vi "Init MemberTable.vi"(8 "error in (no error)":errorcluster, 9 "SheetName(\"\")":string, 10 "Path":path, 11 "TimeTable in":refnum<class "TimeTable.lvclass">) -> (0 "error out":errorcluster, 3 "TimeTable out":refnum<class "TimeTable.lvclass">)   [LabVIEW 2015, in "Member_Actor.lvlib" / "TimeTable.lvclass"]
uses:
  TimeTable.lvclass
  TimeTable.lvclass/TimeTable.ctl
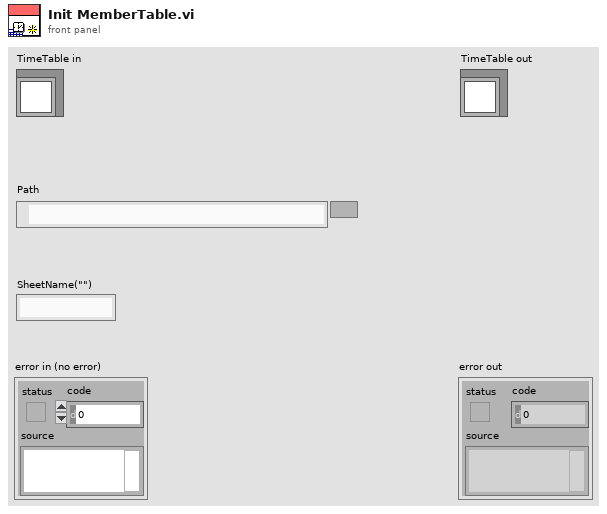
[diagram p1: front panel]
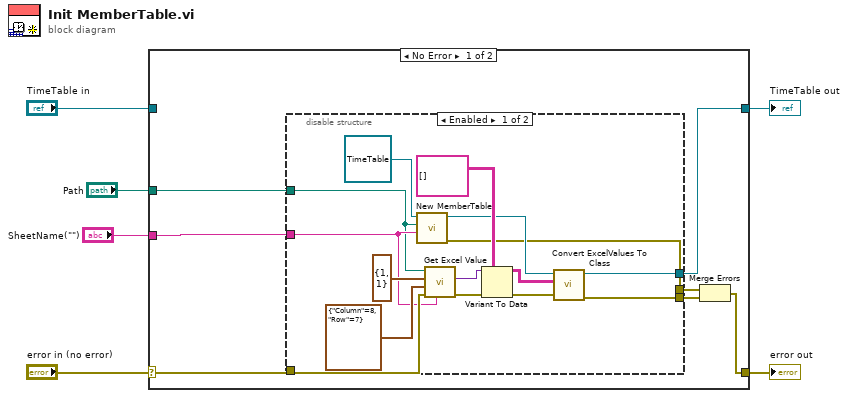
[diagram p0: block diagram]
diagram:
  n1 = case shown="No Error" "error in (no error)" {
    selector: "error in (no error)" -> [w10 w30]
    tunnel: [w12 w30] -> w5
    tunnel: [w11 w29] -> w3
    tunnel: "TimeTable in" -> [_ w29]
    tunnel: "Path" -> [w8 _]
    tunnel: "SheetName(\"\")" -> [w9 _]
    frame No Error {
      n2 = disable-structure shown="Enabled" {
        disable-tunnel: [w28 _] -> w13
        disable-tunnel: [w27 _] -> w11
        disable-tunnel: w10 -> [w20 _]
        disable-tunnel: w9 -> [w16 _]
        disable-tunnel: w8 -> [w15 _]
        disable-tunnel: [w14 _] -> w7
        frame Enabled {
          n3 = call "New MemberTable.vi"("SheetName(\"\")"=w16, "Path"=w15, "MemberTable in"=refnum<class "TimeTable.lvclass"> refnum) -> ("error out"=w14:errorcluster, "MemberTable out"=w17:refnum<class "TimeTable.lvclass">)  [unwired: 7 in]
          n4 = call "Get Excel Value.vi"("SheetName(\"\")"=w16, "error in (no error)"=w20, "End"=cluster{"Column":i32, "Row":i32} {"Column"=8, "Row"=7}, "Start"=cluster{"Column":i32, "Row":i32} {"Column"=1, "Row"=1}, "path"=w15) -> ("error out"=w26:errorcluster, "Excel_Value"=w24:variant)  [unwired: 5 in]
          n5 = Variant To Data(error in=w26, type=string[][] [], Variant=w24) -> (data=w18:string[][], error out=w19:errorcluster)
          n6 = call "Convert ExcelValues To Class.vi"("error in (no error)"=w19, "Excel Value(\"\")"=w18, "MemberTable in"=w17) -> ("error out"=w28:errorcluster, "MemberTable out"=w27:refnum<class "TimeTable.lvclass">)  [unwired: 7 in]
        }
        frame Disabled {
        }
      }
      n7 = Merge Errors(w7, w13) -> (w12:errorcluster)
    }
    frame Error {
    }
  }
  "error out" <- w5
  "TimeTable out" <- w3
